vi "Tosca-Multirig.vi"() -> ()   [LabVIEW 2020]
uses:
  epl-vi-lib/Utility VIs/Math VIs/LinSpace (x0-dx-npts).vi
panel:
  out "Status":string="Starting..."
  in  "Settings Button":bool
  in  "Start Button":bool
  in  "RigList":i32[](listbox)
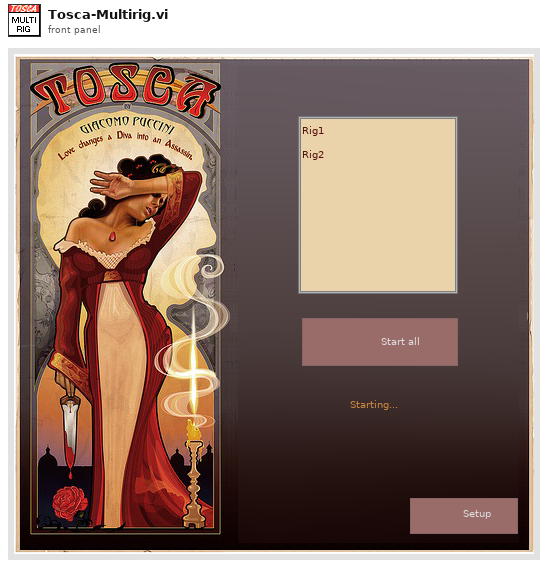
[diagram p1: front panel]
types:
  T1 = enum8{"Enabled", "Disabled", "Disabled and Grayed Out"}
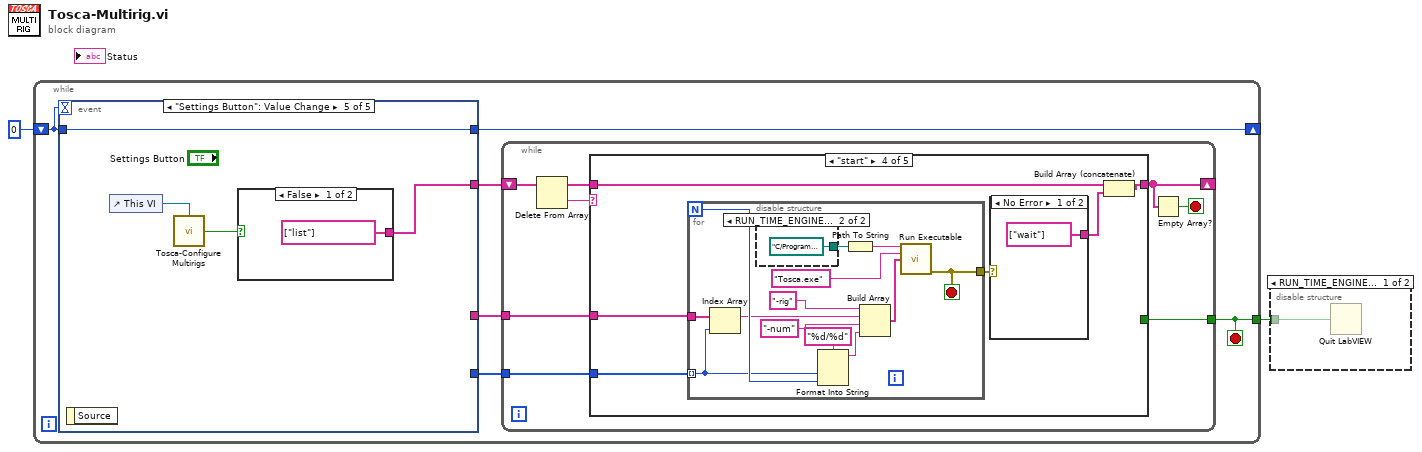
[diagram p0: block diagram]
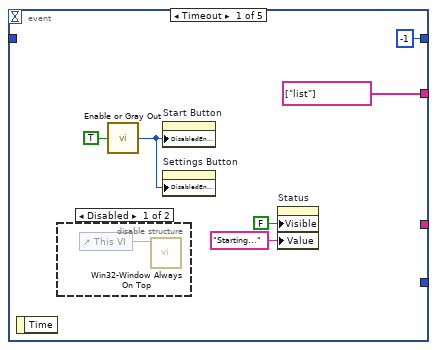
[diagram p2: hidden frame]
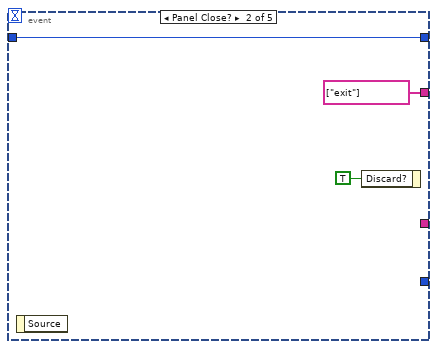
[diagram p4: hidden frame]
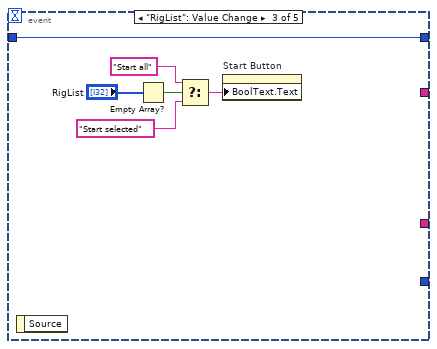
[diagram p5: hidden frame]
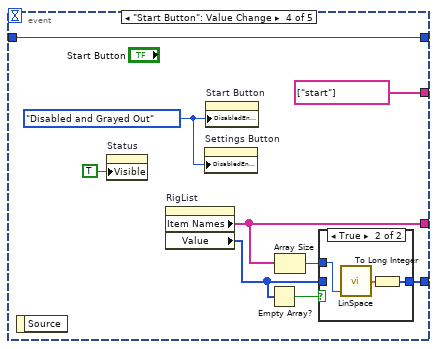
[diagram p6: hidden frame]
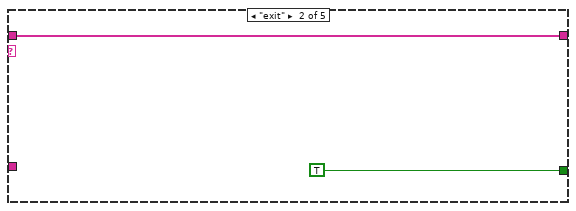
[diagram p10: hidden frame]
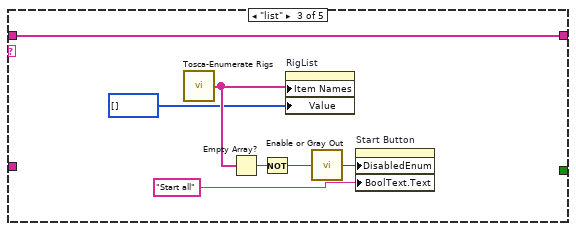
[diagram p11: hidden frame]
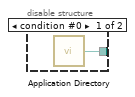
[diagram p12: hidden frame]
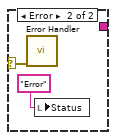
[diagram p13: hidden frame]
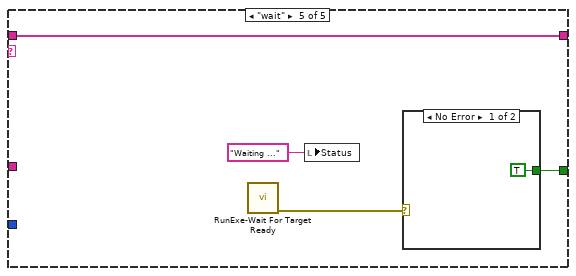
[diagram p14: hidden frame]
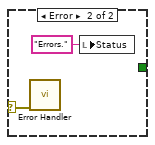
[diagram p15: hidden frame]
diagram:
  n1 = while {
    shift-right: [w7] -> _
    shift-left: 0 -> [w8]
    tunnel: [w5] -> w1
    stop <- w5 stop-if-true
    n2 = event shown="[4] \"Settings Button\": Value Change" {
      selector: _ -> [_ _ _ _ _]
      dyn-events: _ -> [_ _ _ _ _]
      timeout: w8 -> [_ _ _ _ _]
      tunnel: w8 -> [_ w18 w24 w33 w41]
      tunnel: [-1 w18 w24 w33 w41] -> w7
      tunnel: [string[] ["list"] string[] ["exit"] _ string[] ["start"] w39] -> w6
      tunnel: [_ _ _ w26 _] -> w4
      tunnel: [_ _ _ w28 _] -> w3
      event Timeout {
        n3 = event-data() -> ()  [unwired: 1 in, 1 out]
        n4 = disable-structure shown="Disabled" {
          frame Disabled {
            n5 = control-ref of="This VI"() -> (w15:refnum<vi>)
            n6 = call "Win32-Window Always On Top.vi"("VI reference"=w15) -> ()  [unwired: 10 in, 1 out]
          }
          frame Enabled {
          }
        }
        n7 = call "Enable or Gray Out.vi"("Boolean"=TRUE) -> ("Disabled"=w10:T1)
        n8 = property on="Start Button" class="Bool"("DisabledEnum"=w10) -> ()  [unwired: 2 in, 2 out]
        n9 = property on="Settings Button" class="Bool"("DisabledEnum"=w10) -> ()  [unwired: 2 in, 2 out]
        n10 = property on="Status" class="Str"("Visible"=FALSE, "Value"="Starting..." ("Loading")) -> ()  [unwired: 2 in, 2 out]
      }
      event Panel Close? {
        n11 = event-data() -> ()  [unwired: 1 in, 1 out]
        n12 = event-data("Discard?"=TRUE) -> ()  [unwired: 1 in, 1 out]
      }
      event "RigList": Value Change {
        n13 = event-data() -> ()  [unwired: 1 in, 1 out]
        n14 = Empty Array?(array="RigList") -> (empty?=w22:bool)
        n15 = Select(t="Start all", s=w22, f="Start selected" ("Boolean Text.Text")) -> (s? t:f=w19:string)
        n16 = property on="Start Button" class="Bool"("BoolText.Text"=w19) -> ()  [unwired: 2 in, 2 out]
      }
      event "Start Button": Value Change {
        w32 = T1."Disabled and Grayed Out" ("Disabled")
        n17 = event-data() -> ()  [unwired: 1 in, 1 out]
        n18 = property on="Status" class="Str"("Visible"=TRUE) -> ()  [unwired: 2 in, 2 out]
        n19 = property on="RigList" class="LstBox (strict)"() -> ("Item Names"=w26:string[], "Value"=w27:i32[])  [unwired: 2 in, 2 out]
        n20 = property on="Settings Button" class="Bool"("DisabledEnum"=w32) -> ()  [unwired: 2 in, 2 out]
        n21 = property on="Start Button" class="Bool"("DisabledEnum"=w32) -> ()  [unwired: 2 in, 2 out]
        n22 = Empty Array?(array=w27) -> (empty?=w29:bool)
        n23 = Array Size(array=w26) -> (size(s)=w25:i32)
        n24 = case shown="True" w29 {
          tunnel: [w34 w35] -> w28
          tunnel: w27 -> [w34 _]
          tunnel: w25 -> [_ w36]
          frame False {
          }
          frame True {
            n25 = call-poly "LinSpace.vi"("npts"=w36) -> ("Array"=w37:dbl[])  [unwired: 3 in, 1 out]
            n26 = To Long Integer(number=w37) -> (32bit integer=w35:i32[])
          }
        }
      }
      event "Settings Button": Value Change {
        n27 = event-data() -> ()  [unwired: 1 in, 1 out]
        n28 = control-ref of="This VI"() -> (w38:refnum<vi>)
        n29 = call "Tosca-Configure Multirigs.vi"("Parent VI"=w38) -> ("Canceled?"=w40:bool)  [unwired: 14 in]
        n30 = case shown="False" w40 {
          tunnel: [string[] ["list"] _] -> w39
          frame False {
          }
          frame True {
          }
        }
      }
    }
    n31 = while {
      shift-right: [w47] -> _
      shift-left: w6 -> [w50]
      tunnel: [w45] -> w5
      tunnel: w4 -> [w44]
      tunnel: w3 -> [w43]
      stop <- w46 stop-if-true
      n32 = Delete From Array(array=w50) -> (deleted portion=w48:string, array with subset deleted=w49:string[])  [unwired: 2 in]
      n33 = case shown="\"start\"" w48 {
        tunnel: w49 -> [w51 w53 w60 w66 w88]
        tunnel: [w51 w53 w60 w64 w88] -> w47
        tunnel: [_ TRUE _ _ w86] -> w45
        tunnel: w44 -> [_ _ _ w62 _]
        tunnel: w43 -> [_ _ _ w61 _]
        frame "", Default {
        }
        frame "exit" {
        }
        frame "list" {
          n34 = call "Tosca-Enumerate Rigs.vi"() -> ("Rigs"=w55:string[])  [unwired: 15 in]
          n35 = Empty Array?(array=w55) -> (empty?=w56:bool)
          n36 = Not(x=w56) -> (.not. x?=w57:bool)
          n37 = property on="RigList" class="LstBox (strict)"("Item Names"=w55, "Value"=i32[] [] ("RigList")) -> ()  [unwired: 2 in, 2 out]
          n38 = call "Enable or Gray Out.vi"("Boolean"=w57) -> ("Disabled"=w58:T1)
          n39 = property on="Start Button" class="Bool"("DisabledEnum"=w58, "BoolText.Text"="Start all" ("Boolean Text.Text")) -> ()  [unwired: 2 in, 2 out]
        }
        frame "start" {
          n40 = for {
            N -> [w69]
            tunnel: w62 -> [w76]
            tunnel: [w77] -> w65
            tunnel: w61 -> [w67] mode=indexing
            stop <- w77 stop-if-true
            n41 = Index Array(array=w76, index=w67) -> (element=w68:string)
            n42 = disable-structure shown="RUN_TIME_ENGINE==False" {
              disable-tunnel: [w80 path "C:/Program Files (x86)/EPL/Tosca/V2984"] -> w79
              frame condition #0 {
                n43 = call <vilib>:"Application Directory.vi"() -> ("Application Directory"=w80:path)
              }
              frame condition #1 (active) {
              }
            }
            n44 = Format Into String(format string="%d/%d", w67, w69) -> (resulting string=w70:string)  [unwired: 2 in, 1 out]
            n45 = Path To String(path=w79) -> (string=w78:string)
            n46 = Build Array("-rig" ("element"), w68, "-num" ("element"), w70) -> (w73:string[])
            n47 = call "Run Executable.vi"("Folder"=w78, ".EXE name"="Tosca.exe" ("name or relative path"), "args"=w73) -> ("error out"=w77:errorcluster)  [unwired: 12 in]
          }
          n48 = case shown="No Error" w65 {
            selector: w65 -> [_ w84]
            tunnel: [string[] ["wait"] _] -> w63
            frame No Error {
            }
            frame Error {
              n49 = call "Error Handler.vi"("error in (no error)"=w84) -> ()  [unwired: 13 in, 2 out]
              n50 = local write "Status"("Error" ("Loading")) -> ()
            }
          }
          n51 = Build Array (concatenate)(w66, w63) -> (w64:string[])
        }
        frame "wait" {
          n52 = call "RunExe-Wait For Target Ready.vi"() -> ("error out"=w87:errorcluster)  [unwired: 15 in]
          n53 = local write "Status"("Waiting ..." ("Status")) -> ()
          n54 = case shown="No Error" w87 {
            selector: w87 -> [_ w91]
            tunnel: [TRUE _] -> w86
            frame No Error {
            }
            frame Error {
              n55 = call "Error Handler.vi"("error in (no error)"=w91) -> ()  [unwired: 13 in, 2 out]
              n56 = local write "Status"("Errors." ("Status")) -> ()
            }
          }
        }
      }
      n57 = Empty Array?(array=w47) -> (empty?=w46:bool)
    }
  }
  n58 = disable-structure shown="RUN_TIME_ENGINE==True" {
    disable-tunnel: w1 -> [w92 _]
    frame condition #0 {
      n59 = Quit LabVIEW(quit? (T)=w92) -> ()
    }
    frame condition #1 (active) {
    }
  }
